vi "GenesysPS.contents.vi"() -> ()   [LabVIEW 2014, in "GenesysPS.lvlib"]
uses:
  GenesysPS.lvlib
panel:
  out "error out":errorcluster
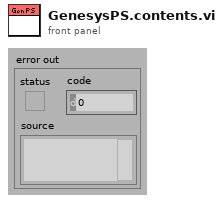
[diagram p1: front panel]
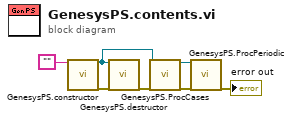
[diagram p0: block diagram]
diagram:
  n1 = call "GenesysPS.constructor.vi"("name"="") -> ("i ref out"=w5:refnum<vi>, "error out"=w4:errorcluster)  [unwired: 16 in, 1 out]
  n2 = call "GenesysPS.destructor.vi"("i ref in"=w5, "error in (no error)"=w4) -> ("error out"=w3:errorcluster)  [unwired: 17 in]
  n3 = call "GenesysPS.ProcCases.vi"("i ref in"=w5, "error in (no error)"=w3) -> ("i ref out"=w7:refnum<vi>, "error out"=w2:errorcluster)  [unwired: 15 in, 1 out]
  n4 = call "GenesysPS.ProcPeriodic.vi"("i ref in"=w7, "error in (no error)"=w2) -> ("error out"=→"error out":errorcluster)  [unwired: 15 in, 2 out]
